vi "LASER_Open.vi"(6 "error in":errorcluster, 9 "Lumencor Com Port":u32) -> (0 "error out":errorcluster)   [LabVIEW 2010]
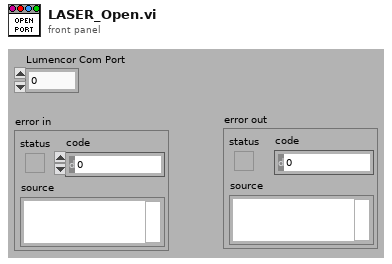
[diagram p1: front panel]
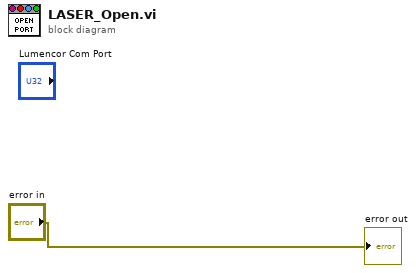
[diagram p0: block diagram]
diagram:
  "error out" <- "error in"
